vi "OCR Get Names2.vi"(7 "error in":errorcluster, 10 "SS Path":path=path "c:/PokerSS/SS.png") -> (0 "Error Out":errorcluster, 3 "All Players Names":string[](array[string]))   [LabVIEW 2015]
uses:
  <vilib>/vision/NI_Vision_Development_Module.lvlib
panel:
  in  "ROI Names":T1(array[cluster])=[{"Global Rectangle"=[1069, 478, 1168, 495], "Contours"=[{"ID"=enum."External", "Type"=3, "Coordinates"=[1069, 478, 1168, 495]}]}, {"Global Rectangle"=[1248, 519, 1366, 535], "Contours"=[{"ID"=enum."External", "Type"=3, "Coordinates"=[1248, 519, 1366, 535]}]}, {"Global Rectangle"=[1387, 681, 1506, 696], "Contours"=[{"ID"=enum."External", "Type"=3, "Coordinates"=[1387, 681, 1506, 696]}]}, {"Global Rectangle"=[1255, 819, 1378, 838], "Contours"=[{"ID"=enum."External", "Type"=3, "Coordinates"=[1255, 819, 1378, 838]}]}, {"Global Rectangle"=[1028, 852, 1145, 868], "Contours"=[{"ID"=enum."External", "Type"=3, "Coordinates"=[1028, 852, 1145, 868]}]}, {"Global Rectangle"=[758, 853, 874, 871], "Contours"=[{"ID"=enum."External", "Type"=3, "Coordinates"=[758, 853, 874, 871]}]}, {"Global Rectangle"=[539, 820, 663, 837], "Contours"=[{"ID"=enum."External", "Type"=3, "Coordinates"=[539, 820, 663, 837]}]}, {"Global Rectangle"=[389, 674, 500, 690], "Contours"=[{"ID"=enum."External", "Type"=3, "Coordinates"=[389, 674, 500, 690]}]}, {"Global Rectangle"=[523, 517, 648, 536], "Contours"=[{"ID"=enum."External", "Type"=3, "Coordinates"=[523, 517, 648, 536]}]}, {"Global Rectangle"=[718, 479, 831, 496], "Contours"=[{"ID"=enum."External", "Type"=3, "Coordinates"=[718, 479, 831, 496]}]}]
  out "Image Out":T2(plugin-control)
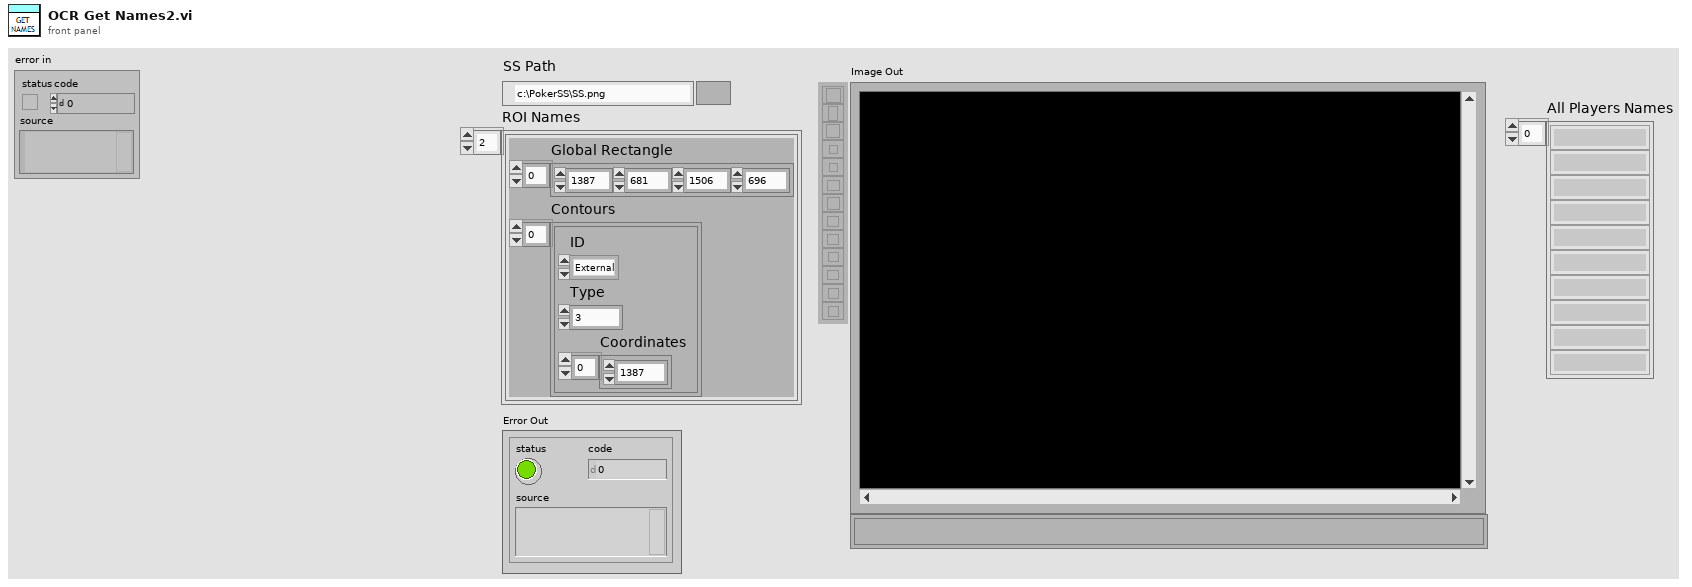
[diagram p1: front panel]
types:
  T1 = cluster{"Global Rectangle":i32[], "Contours":cluster{"ID":enum32{"External", "Internal"}, "Type":u32, "Coordinates":i32[]}[]}[]
  T2 = typedef "IMAQ Image.ctl" = refnum<image>
  T3 = cluster{"Threshold Data":cluster{"Method":enum16{"Fixed Range", "Uniform", "Linear", "Non Linear", "Local", "Color"}, "Looking for":u32, "Color Mode":u32, "Kernel Size":cluster{"Width":i32, "Height":i32}, "Ranges":cluster{"Min":i32, "Max":i32}[]}, "Reject Border":bool, "Number Of Erosions":i32, "Size & Spacing":cluster{"Segment Algorithm":u16, "Min Bounding Rect Width":i32, "Max Bounding Rect Width":i32, "Min Bounding Rect Height":i32, "Max Bounding Rect Height":i32, "Min Character Size":i32, "Max Character Size":i32, "Min Char Spacing":i32, "Max Horiz Element Spacing":i32, "Max Vert Element Spacing":i32, "Max Space Distance":i32}, "Read Options":cluster{"Read Strategy":i32, "Read Resolution":i32, "Scale Dependant":bool, "Aspect Ratio":i32, "Acceptance Level":i32, "Substitution Character":string, "MultiLine":bool}, "Valid Characters":cluster{"Pre-defined characters":i32, "User-defined characters":string}[], "Use Text Pattern":bool, "Orientation":u32, "# Lines Expected":u32, "Number of Blocks":i32}
  T4 = typedef "Image Type" = u32
  T5 = typedef "IMAQ OCR Session.ctl" = refnum<k1>
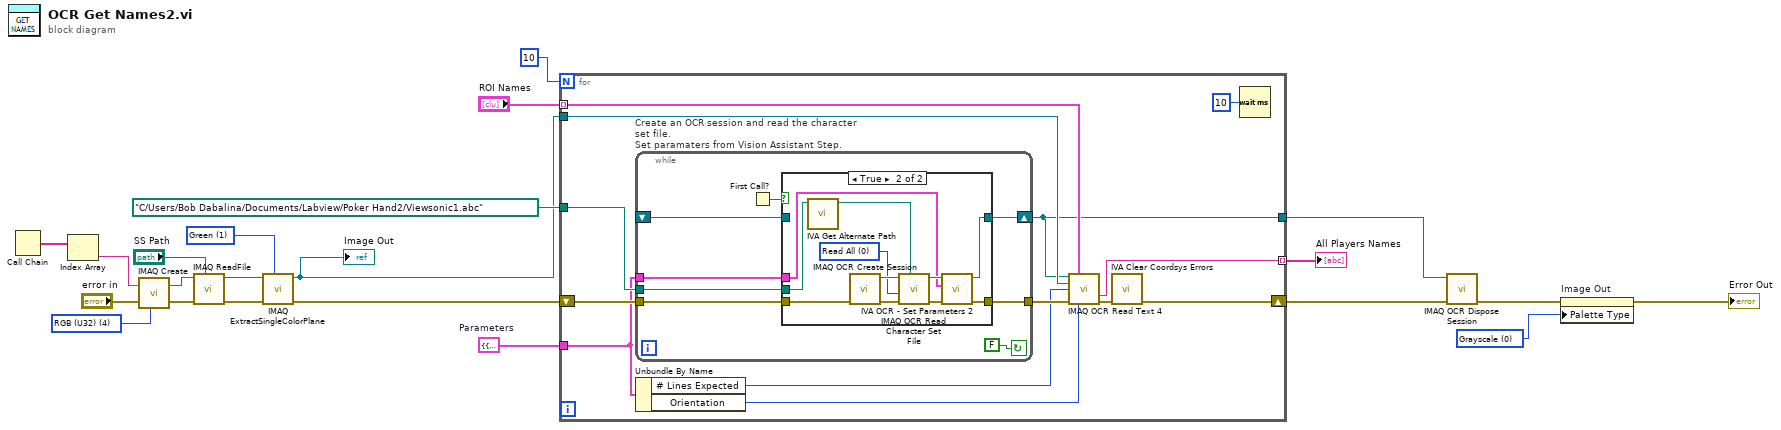
[diagram p0: block diagram]
diagram:
  w6 = u32 0 items=["Grayscale", "Binary", "Gradient", "Rainbow", "Temperature", "User Defined", "Binary 16 Bit", "Gradient 16 Bit", "Rainbow 16 Bit", "Temperature 16 Bit", "User Defined 16 Bit"] ("Palette Type")
  w11 = T3 {"Threshold Data"={"Method"=enum."Linear", "Looking for"=1, "Color Mode"=0, "Kernel Size"={"Width"=32, "Height"=32}, "Ranges"=[{"Min"=1, "Max"=255}]}, "Reject Border"=TRUE, "Number Of Erosions"=0, "Size & Spacing"={"Segment Algorithm"=0, "Min Bounding Rect Width"=2, "Max Bounding Rect Width"=7, "Min Bounding Rect Height"=2, "Max Bounding Rect Height"=65536, "Min Character Size"=4, "Max Character Size"=5555, "Min Char Spacing"=1, "Max Horiz Element Spacing"=1, "Max Vert Element Spacing"=0, "Max Space Distance"=65536}, "Read Options"={"Read Strategy"=1, "Read Resolution"=2, "Scale Dependant"=FALSE, "Aspect Ratio"=400, "Acceptance Level"=700, "Substitution Character"="?", "MultiLine"=FALSE}, "Valid Characters"=[], "Use Text Pattern"=FALSE, "Orientation"=0, "# Lines Expected"=0, "Number of Blocks"=4}  # Parameters
  w15 = 1 items=["Red", "Green", "Blue", "Hue", "Saturation", "Luminance", "Value", "Intensity"] ("Color Plane")
  w16 = T4 4 items=["Grayscale (U8)", "Grayscale (I16)", "Grayscale (SGL)", "Complex (CSG)", "RGB (U32)", "HSL (U32)", "RGB (U64)", "Grayscale (U16)"] ("Image Type")
  n1 = Call Chain() -> (call chain=w18:string[])
  n2 = Index Array(array=w18) -> (element=w17:string)  [unwired: 1 in]
  n3 = call "IMAQ Create"("Image Name"=w17, "Image Type"=w16, "error in (no error)"="error in") -> ("New Image"=w21:T2, "error out"=w20:errorcluster)  [unwired: 1 in, 1 out]
  n4 = call "IMAQ ReadFile"("File Path"="SS Path", "error in (no error)"=w20, "Image"=w21) -> ("error out"=w22:errorcluster, "Image Out"=w14:T2)  [unwired: 2 in, 5 out]
  n5 = call "IMAQ ExtractSingleColorPlane"("Color Plane"=w15, "error in (no error)"=w22, "Image Src"=w14) -> ("error out"=w13:errorcluster, "Image Dst Out"=w10:T2)  [unwired: 1 in, 6 out]
  "Image Out" <- w10
  n6 = for {
    N: 10 -> [_]
    tunnel: path "C:/Users/Bob Dabalina/Documents/Labview/Poker Hand2/Viewsonic1.abc" ("File Path") -> [w34]
    tunnel: w11 -> [w33]
    tunnel: w10 -> [w29]
    shift-right: [w26] -> w3
    shift-left: w13 -> [w35]
    tunnel: "ROI Names" -> [w28] mode=indexing
    tunnel: [w25] -> w4 mode=indexing
    tunnel: [w24] -> w1
    n7 = while "Create an OCR session and read the character set file.\nSet paramaters from Vision Assistant Step." {
      shift-right: [w40] -> w24
      shift-left: _ -> [w39]
      tunnel: w35 -> [w42]
      tunnel: w33 -> [w38]
      tunnel: w34 -> [w37]
      tunnel: [w36] -> w32
      stop <- FALSE continue-if-true
      n8 = First Call?() -> (First Call?: T/F=w41:bool)
      n9 = case shown="True" w41 {
        tunnel: w37 -> [_ w49]
        tunnel: w42 -> [w44 w53]
        tunnel: [w45 w51] -> w40
        tunnel: [w44 w50] -> w36
        tunnel: w38 -> [_ w46]
        tunnel: w39 -> [w45 _]
        frame False {
        }
        frame True {
          w54 = 0 items=["Read All", "Read Character Set Only", "Read Properties Only"] ("Read Options")
          n10 = call <vilib>:"IVA Get Alternate Path.vi"("Path In"=w49) -> ("Path Out"=w48:path)  [unwired: 10 out]
          n11 = call "IMAQ OCR Create Session"("error in (no error)"=w53) -> ("error out"=w55:errorcluster, "IMAQ OCR Session"=w56:T5)  [unwired: 9 out]
          n12 = call "IMAQ OCR Read Character Set File"("File Path"=w48, "error in (no error)"=w55, "Read Options"=w54, "IMAQ OCR Session"=w56) -> ("error out"=w52:errorcluster, "IMAQ OCR Session (dup)"=w47:T5)  [unwired: 1 in, 5 out]
          n13 = call <vilib>:"IVA OCR - Set Parameters 2.vi"("error in (no error)"=w52, "Parameters"=w46, "IMAQ OCR Session"=w47) -> ("error out"=w50:errorcluster, "IMAQ OCR Session Out"=w51:T5)  [unwired: 7 in]
        }
      }
    }
    n14 = Unbundle By Name(w33) -> ("# Lines Expected"=w30:u32, "Orientation"=w31:u32)
    n15 = call "IMAQ OCR Read Text 4"("IMAQ OCR Session"=w24, "ROI Descriptor"=w28, "Image"=w29, "Number of Lines Requested"=w30, "error in (no error)"=w32, "Orientation"=w31) -> ("Read String"=w25:string, "error out"=w27:errorcluster)  [unwired: 8 out]
    n16 = call <vilib>:"IVA Clear Coordsys Errors.vi"("error in (no error)"=w27) -> ("error out"=w26:errorcluster)  [unwired: 10 in]
    n17 = Wait (ms)(milliseconds to wait=u32 10) -> ()  [unwired: 1 out]
  }
  "All Players Names" <- w4
  n18 = call "IMAQ OCR Dispose Session"("error in (no error)"=w3, "IMAQ OCR Session"=w1) -> ("error out"=w2:errorcluster)  [unwired: 9 in]
  n19 = property on="Image Out" class="ImageControl"(error in=w2, "Palette Type"=w6) -> (error out=→"Error Out":errorcluster)  [unwired: 1 in, 1 out]
